vi "Construct.vi"(8 "port":i32, 10 "station":u8, 11 "ipAddress":string) -> (3 "MelsecMcNet out":refnum<class "Inovance5UTcp.lvclass">)   [LabVIEW 2020, in "HslCommunication.lvlib" / "Inovance5UTcp.lvclass"]
uses:
  Inovance5UTcp.lvclass
  Inovance5UTcp.lvclass/Inovance5UTcp.ctl
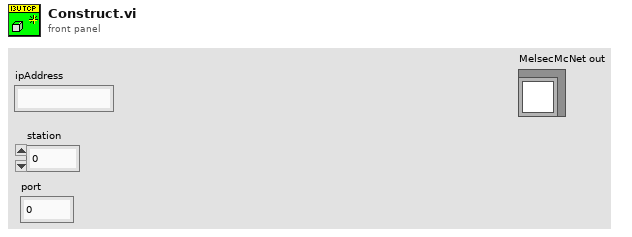
[diagram p1: front panel]
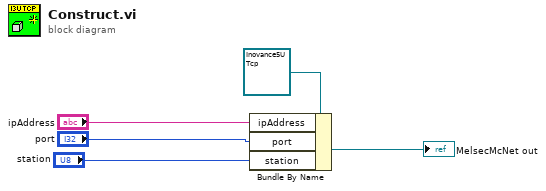
[diagram p0: block diagram]
diagram:
  n1 = Bundle By Name(cluster=refnum<class "Inovance5UTcp.lvclass"> refnum ("MelsecMcNet in"), "ipAddress"="ipAddress", "port"="port", "station"="station") -> (→"MelsecMcNet out":refnum<class "Inovance5UTcp.lvclass">)
